vi "GetWindowSurface.vi"(8 "No Error":errorcluster, 11 "Window [SDL_Window *]":i64) -> (0 "Error Out":errorcluster, 3 "Surface [SDL_Surface *]":i64)   [LabVIEW 2024, in "SDL3.lvlib" / "Video.lvlib"]
doc: "<B>Summary</B>\nGet the SDL surface associated with the window.\n\n<B>Remarks</B>\nA new surface will be created with the optimal format for the window, if necessary. This surface will be freed when the window is destroyed. Do not free this surface.\n\nThis surface will be invalidated if the window is resized. After resizing a window this function must be called again to return a valid surface.\n\nYou may not combine this with 3D or the rendering API on this window.\n\nThis function is affected by <B>SDL_HINT_FRAMEBUFFER_ACCELERATION</B>."
uses:
  Video.lvlib
  Error/Error.lvlib
  Lib/SDL3-32.dll
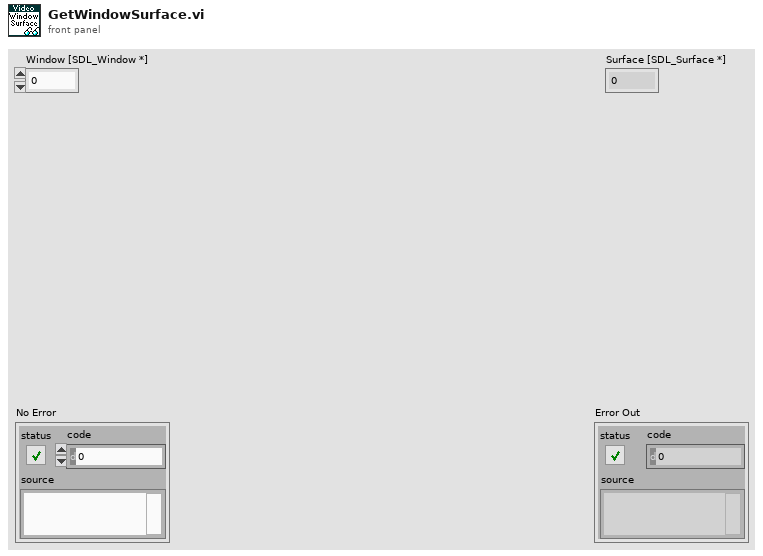
[diagram p1: front panel]
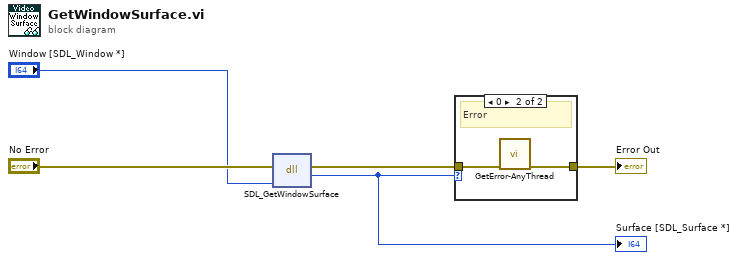
[diagram p0: block diagram]
diagram:
  n1 = dll-call lib="C:/Users/Thomas/Documents/Projects/LV-SDL3/Lib/SDL3-*.*" fn="SDL_GetWindowSurface"(error in="No Error", "window"="Window [SDL_Window *]") -> (error out=w2:errorcluster, "return type"=w1:i64)  [unwired: 3 in, 1 out]
  "Surface [SDL_Surface *]" <- w1
  n2 = case shown="0" w1 {
    tunnel: w2 -> [w6 w8]
    tunnel: [w6 w7] -> w4
    frame Default {
      # "Ok"
    }
    frame 0 {
      # "Error"
      n3 = call "GetError-AnyThread.vi"("No Error"=w8) -> ("Error Out"=w7:errorcluster)  [unwired: 10 in]
    }
  }
  "Error Out" <- w4
